vi "Setup.vi"(8 "error in (no error)":errorcluster, 11 "Mock Process Test In":refnum<class "Mock Process Test.lvclass">) -> (0 "error out":errorcluster, 3 "Mock Process Test Out":refnum<class "Mock Process Test.lvclass">)   [LabVIEW 2020, in "Mock Process Test.lvclass"]
uses:
  Mock Process Test.lvclass
  C:/Git/astemes-triarc-framework/source/Framework Test/Base Class Test/Base Test.lvclass
  source/Framework Test Suite/Mock Process/Mock Process.lvclass
  C:/Git/astemes-triarc-framework/source/Framework/Base/Base.lvclass
  source/Framework Test Suite/Base Class Test/Base Test.lvclass/Base Test.ctl
  source/Framework Test Suite/Base Class Test/Base Test.lvclass
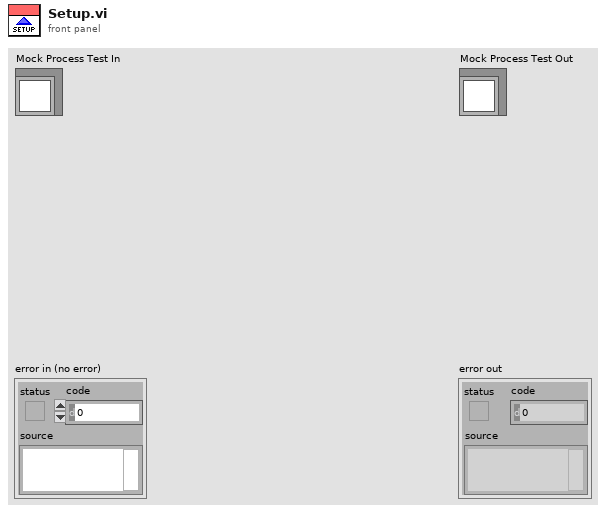
[diagram p1: front panel]
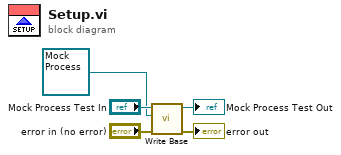
[diagram p0: block diagram]
diagram:
  n1 = call "Write Base.vi"("error in (no error)"="error in (no error)", "Base"=refnum<class "Mock Process.lvclass"> refnum ("Mock Process.lvclass"), "Base Class Test In"="Mock Process Test In") -> ("error out"=→"error out":errorcluster, "Base Class Test Out"=→"Mock Process Test Out":refnum<class "Mock Process Test.lvclass">)  [unwired: 7 in]
